vi "Post-Build Custom Action.vi"(10 "Variant":variant) -> (0 "error out":errorcluster)   [LabVIEW 2019]
uses:
  <userlib>/LevyLab/Build Support/PostBuildSupport/PostBuildSupport.lvclass
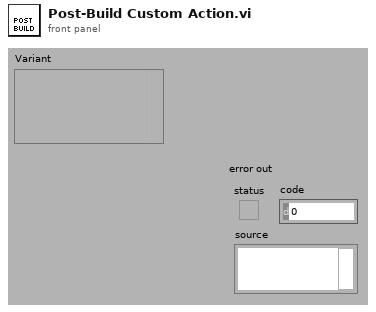
[diagram p1: front panel]
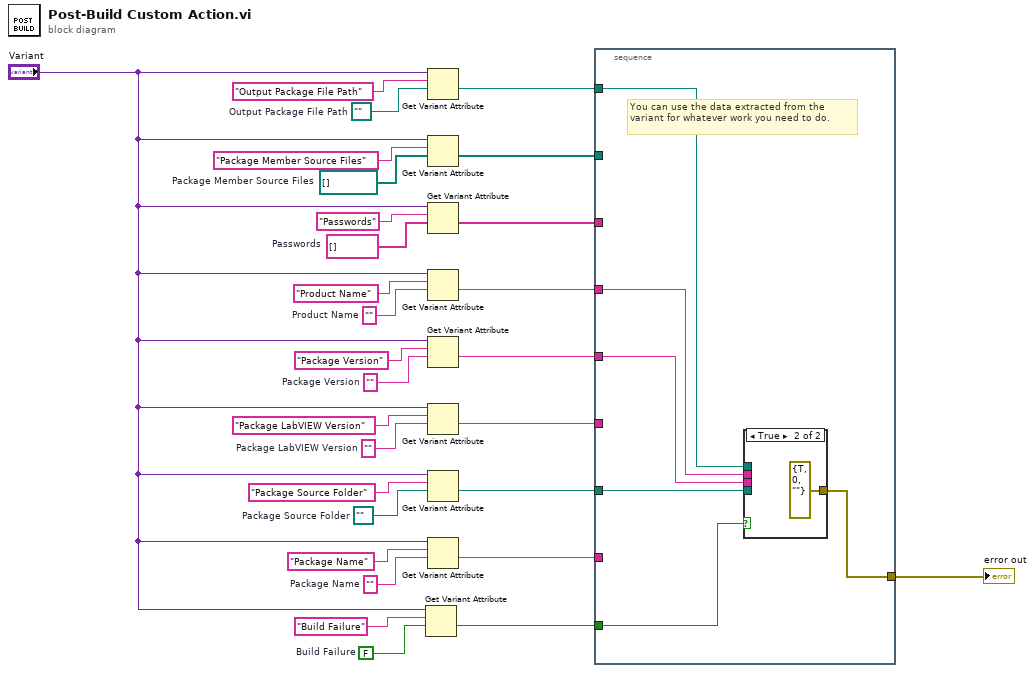
[diagram p0: block diagram]
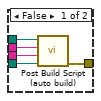
[diagram p2: hidden frame]
diagram:
  w4 = FALSE  # Build Failure
  w14 = path ""  # Package Source Folder
  w15 = ""  # Package Name
  w18 = ""  # Package LabVIEW Version
  w20 = ""  # Package Version
  w22 = ""  # Product Name
  w24 = string[] []  # Passwords
  w26 = path[] []  # Package Member Source Files
  w28 = path ""  # Output Package File Path
  n1 = Get Variant Attribute(Variant="Variant", name="Build Failure", default value (empty Variant)=w4) -> (value=w2:bool)  [unwired: 1 in, 3 out]
  n2 = Get Variant Attribute(Variant="Variant", name="Output Package File Path", default value (empty Variant)=w28) -> (value=w13:path)  [unwired: 1 in, 3 out]
  n3 = Get Variant Attribute(Variant="Variant", name="Package Member Source Files", default value (empty Variant)=w26) -> (value=w12:path[])  [unwired: 1 in, 3 out]
  n4 = Get Variant Attribute(Variant="Variant", name="Passwords", default value (empty Variant)=w24) -> (value=w11:string[])  [unwired: 1 in, 3 out]
  n5 = Get Variant Attribute(Variant="Variant", name="Product Name", default value (empty Variant)=w22) -> (value=w10:string)  [unwired: 1 in, 3 out]
  n6 = Get Variant Attribute(Variant="Variant", name="Package Version", default value (empty Variant)=w20) -> (value=w9:string)  [unwired: 1 in, 3 out]
  n7 = Get Variant Attribute(Variant="Variant", name="Package LabVIEW Version", default value (empty Variant)=w18) -> (value=w8:string)  [unwired: 1 in, 3 out]
  n8 = Get Variant Attribute(Variant="Variant", name="Package Source Folder", default value (empty Variant)=w14) -> (value=w7:path)  [unwired: 1 in, 3 out]
  n9 = Get Variant Attribute(Variant="Variant", name="Package Name", default value (empty Variant)=w15) -> (value=w6:string)  [unwired: 1 in, 3 out]
  n10 = stacked-sequence {
    tunnel: w13 -> [w35]
    tunnel: w12 -> [_]
    tunnel: w11 -> [_]
    tunnel: w10 -> [w34]
    tunnel: w9 -> [w33]
    tunnel: w8 -> [_]
    tunnel: w7 -> [w32]
    tunnel: w6 -> [_]
    tunnel: w2 -> [w31]
    tunnel: [w30] -> w1
    frame #0 {
      # "You can use the data extracted from the variant for whatever work you need to do."
      n11 = case shown="True" w31 {
        tunnel: w35 -> [w40 _]
        tunnel: w34 -> [w39 _]
        tunnel: w33 -> [w38 _]
        tunnel: w32 -> [w37 _]
        tunnel: [w36 errorcluster {"status"=TRUE, "code"=0, "source"=""} ("error out")] -> w30
        frame False {
          n12 = call <userlib>:"Post Build Script (auto build).vi"("Package Source Folder"=w37, "Package Version"=w38, "Product Name"=w39, "Output Package File Path"=w40) -> ("error out"=w36:errorcluster)  [unwired: 7 in]
        }
        frame True {
        }
      }
    }
  }
  "error out" <- w1
